vi "rename custom device xml.vi"(8 "error in (no error)":errorcluster, 10 "User Project":refnum<vi>, 11 "NIVS_CDW_MetaDataObj in":refnum<class "NIVS_ScriptedModuleTemplate_MetaDataObj.lvclass">) -> (0 "error out":errorcluster, 3 "new xml path":path)   [LabVIEW 2014, in "NIVS_ScriptedModuleTemplate_MetaDataObj.lvclass"]
uses:
  NIVS_ScriptedModuleTemplate_MetaDataObj.lvclass
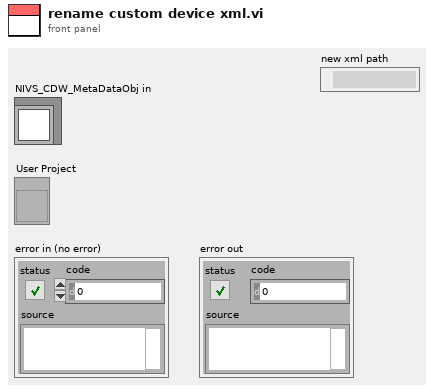
[diagram p1: front panel]
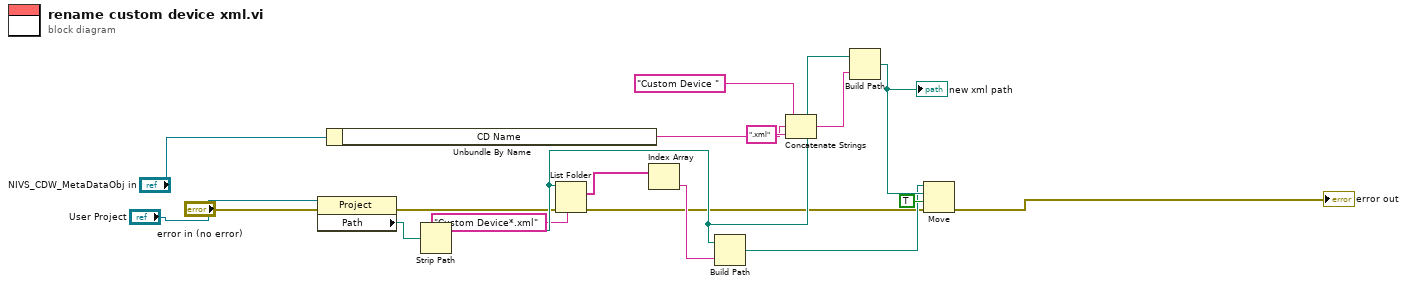
[diagram p0: block diagram]
diagram:
  n1 = property class="Project"(reference="User Project", error in="error in (no error)") -> (error out=w2:errorcluster, "Path"=w4:path)  [unwired: 1 out]
  n2 = Unbundle By Name("NIVS_CDW_MetaDataObj in") -> ("CD Name"=w9:string)
  n3 = Strip Path(path=w4) -> (stripped path=w13:path)  [unwired: 1 out]
  n4 = List Folder(path=w13, pattern="Custom Device*.xml", error in=w2) -> (filenames=w7:string[], error out=w5:errorcluster)  [unwired: 1 in, 2 out]
  n5 = Index Array(array=w7) -> (element=w12:string)  [unwired: 1 in]
  n6 = Build Path(base path=w13, name or relative path=w12) -> (appended path=w16:path)
  n7 = Concatenate Strings("Custom Device " ("string"), w9, ".xml" ("string")) -> (w14:string)
  n8 = Build Path(base path=w13, name or relative path=w14) -> (appended path=w17:path)
  "new xml path" <- w17
  n9 = Move(source path=w16, error in=w5, 9:TRUE ("overwrite (F)"), 10:w17) -> (error out=→"error out":errorcluster)  [unwired: 1 in, 2 out]
